vi "Kommunikation Regler.vi"(8 "error in (no error)":errorcluster caption="Fehler (Eingang, kein Fehler)", 10 "Index":u16, 11 "Steuerung PNS Eingang":refnum<class "Steuerung PNS.lvclass">) -> (0 "error out":errorcluster caption="Fehler (Ausgang)", 2 "Werte":cluster{u16[], u16[]}, 3 "Steuerung PNS Ausgang":refnum<class "Steuerung PNS.lvclass">)   [LabVIEW 2020, in "Steuerung PNS.lvclass"]
doc: "Kommuniziert mit der Steuerung, um die Regler (nach Index) auszulesen und speichert diese im Objekt.\nDie Istwerte werden mit den Sollwerten verglichen und bei Unterschieden die Werte zum schreiben (Adresse/Wert Cluster) werden auch im Objekt gespeichert und gelichzeitig als Output zur Verfügung gestellt.\nHier werden auch die PV Fehler gesetzt (Error Code).\n(automatisch je nach Steuerungstype werden die richtigen Adressen verwendet - durch die transparente SubKlasse)\n(Implementierung des Ist Soll Vergleichs in der jeweiligen SubKlasse)\nRIW"
uses:
  Steuerung PNS.lvclass
  Steuerung PNS.lvclass/Steuerung PNS.ctl
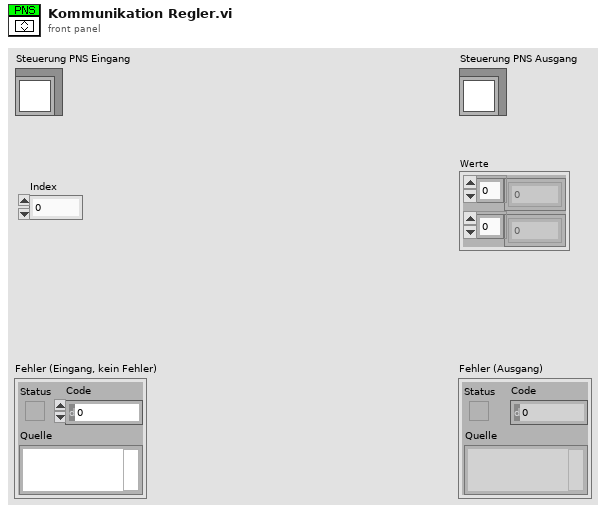
[diagram p1: front panel]
types:
  T1 = typedef "Steuerung PNS.lvclass/Adresse.ctl" = cluster{i32[][], i32}
  T2 = typedef "Steuerung PNS.lvclass/Werte.ctl" = cluster{"Adressen":u16[], "Werte":u16[]}
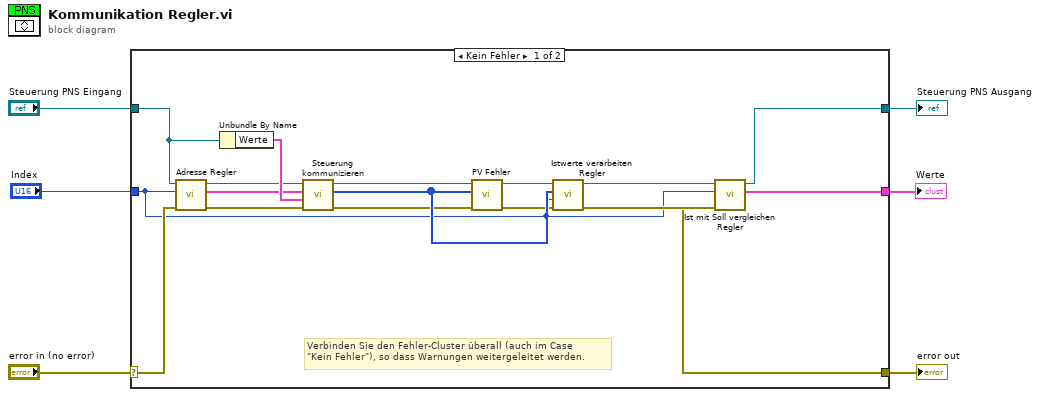
[diagram p0: block diagram]
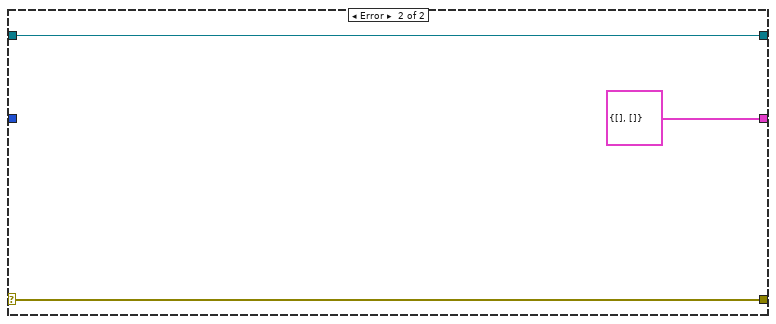
[diagram p2: hidden frame]
diagram:
  n1 = case shown="Kein Fehler" "error in (no error)" {
    selector: "error in (no error)" -> [w16 w26]
    tunnel: [w15 w26] -> w5
    tunnel: [w13 w25] -> w3
    tunnel: "Steuerung PNS Eingang" -> [w14 w25]
    tunnel: "Index" -> [w7 _]
    tunnel: [w12 cluster{u16[], u16[]} {[], []} ("Werte")] -> w1
    frame No Error {
      # "Verbinden Sie den Fehler-Cluster überall (auch im Case\n\"Kein Fehler\"), so dass Warnungen weitergeleitet werden."
      n2 = call-dynamic "Adresse Regler.vi"("error in (no error)"=w16, "Index"=w7, "Steuerung PNS Eingang"=w14) -> ("error out"=w19:errorcluster, "Adressen"=w20:T1, "Steuerung PNS Ausgang"=w21:refnum<class "Steuerung PNS.lvclass">)  [unwired: 6 in]
      n3 = Unbundle By Name(w14) -> ("Werte"=w22:T2)
      n4 = call "Steuerung kommunizieren.vi"("Steuerung PNS Eingang"=w21, "Adressen"=w20, "Werte"=w22, "error in (no error)"=w19) -> ("Steuerung PNS Ausgang"=w11:refnum<class "Steuerung PNS.lvclass">, "Istwerte"=w23:u16[], "error out"=w9:errorcluster)  [unwired: 4 in]
      n5 = call "PV Fehler.vi"("error in (no error)"=w9, "Istwerte"=w23, "Steuerung PNS Eingang"=w11) -> ("error out"=w8:errorcluster, "Steuerung PNS Ausgang"=w10:refnum<class "Steuerung PNS.lvclass">)  [unwired: 7 in]
      n6 = call-dynamic "Istwerte verarbeiten Regler.vi"("error in (no error)"=w8, "Index"=w7, "Istwerte"=w23, "Steuerung PNS Eingang"=w10) -> ("error out"=w17:errorcluster, "Steuerung PNS Ausgang"=w18:refnum<class "Steuerung PNS.lvclass">)  [unwired: 6 in]
      n7 = call-dynamic "Ist mit Soll vergleichen Regler.vi"("error in (no error)"=w17, "Index"=w7, "Steuerung PNS Eingang"=w18) -> ("error out"=w15:errorcluster, "Werte"=w12:cluster{u16[], u16[]}, "Steuerung PNS Ausgang"=w13:refnum<class "Steuerung PNS.lvclass">)  [unwired: 6 in]
    }
    frame Error {
    }
  }
  "error out" <- w5
  "Steuerung PNS Ausgang" <- w3
  "Werte" <- w1
